vi "Write Name Specs.vi"(10 "Name Specs":refnum<class "Name Specs.lvclass">, 11 "_Msg Rescript in":refnum<class "_Msg Rescript.lvclass">) -> (3 "_Msg Rescript out":refnum<class "_Msg Rescript.lvclass">)   [LabVIEW 2025, in "_Msg Rescript.lvlib" / "_Msg Rescript.lvclass"]
uses:
  _Msg Rescript.lvclass
  _Shared/Name Specs/Name Specs.lvclass
  _Msg Rescript.lvclass/_Msg Rescript.ctl
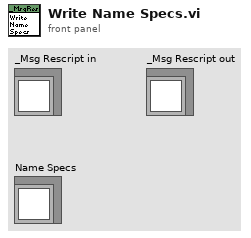
[diagram p1: front panel]
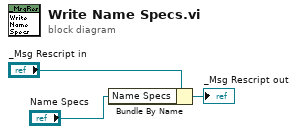
[diagram p0: block diagram]
diagram:
  n1 = Bundle By Name(cluster="_Msg Rescript in", "Name Specs"="Name Specs") -> (→"_Msg Rescript out":refnum<class "_Msg Rescript.lvclass">)
